vi "Main.vi"(11 "Module Admin":refnum<class "Delacor_lib_QMH_Module Admin.lvclass">) -> ()   [LabVIEW 2019, in "MAIN.lvlib"]
doc: "This template is based off of the Queued Message Handler design pattern and the Queued Message Handler project template that ships with LabVIEW.\n\nThe main difference is that the queue is private to this module and communication between modules is performed via Broadcast and Request events.\n\nRequest events are wrapped in public API methods and are handled in the Event Handling Loop (EHL) of this VI. Any module can register for Broadcast events sent by this module. The EHL generates messages based on user interface actions.\n\nThe Message Handling Loop (MHL) processes messages generated by the EHL, or by other messages. The messages are string values, so new messages can be added easily to the Message Cases case structure in the MHL. Each message cluster can also provide an optional value for Message Data, which is a variant that can be converted to whatever message-specific data is required.\n_____\nBased on Delacor QMH Project Template 5.0.0.82."
uses:
  MAIN.lvlib
  <vilib>/Delacor/Delacor QMH/Libraries/Module Admin_class/Delacor_lib_QMH_Module Admin.lvclass
  Module Data--cluster.ctl
  <vilib>/Delacor/Delacor QMH/Libraries/Message Queue_class/Delacor_lib_QMH_Message Queue.lvclass/Delacor_lib_QMH_Message Queue.ctl
  Stop Argument--cluster.ctl
  <vilib>/Delacor/Delacor QMH/Libraries/Module Admin_class/Delacor_lib_QMH_Module Admin.lvclass/Delacor_lib_QMH_Module Admin.ctl
  START HELPER LOOP Argument--cluster.ctl
  STOP HELPER LOOP Argument--cluster.ctl
  SOLICITAR DATOS DE CONEXION Argument--cluster.ctl
  <vilib>/Utility/miscctls.llb/LVPointTypeDef.ctl
  <vilib>/Delacor/Delacor QMH/Libraries/Message Queue_class/Delacor_lib_QMH_Enqueue Message (Single).vi
  <vilib>/Delacor/Delacor QMH/Libraries/Module Admin_class/Delacor_lib_QMH_Get External Launch.vi
  <vilib>/Utility/error.llb/Error Cluster From Error Code.vi
  <vilib>/ErrorRing/Error Ring.xnode
  <vilib>/Delacor/Delacor QMH/Libraries/Message Queue_class/Delacor_lib_QMH_Message Queue.lvclass
panel:
  out "Microcontrolador":string
  out "SE CONECTÓ?":bool
  in  "CONECTAR AL MICRO":bool
  in  "PUERTO DE CONEXIÓN":refnum<visa-resource-name>
  in  "Simulate MHL Error":bool
  in  "Simulate EHL Error":bool
  out "error out":errorcluster
  out "Status":string
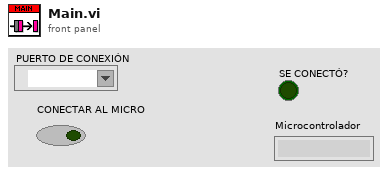
[diagram p1: front panel]
types:
  T1 = typedef "MAIN.lvlib/Request Events--cluster.ctl" = cluster{"Stop Module":refnum<user-event>, "Show Panel":refnum<user-event>, "Hide Panel":refnum<user-event>, "Get Module Execution Status":refnum<user-event>, "Show Diagram":refnum<user-event>, "START HELPER LOOP":refnum<user-event>, "STOP HELPER LOOP":refnum<user-event>, "SOLICITAR DATOS DE CONEXION":refnum<user-event>}
  T2 = typedef "CONEXIÓN CON EL MICRO.lvlib/Broadcast Events--cluster.ctl" = cluster{"Module Did Init":refnum<user-event>, "Status Updated":refnum<user-event>, "Error Reported":refnum<user-event>, "Module Did Stop":refnum<user-event>, "Update Module Execution Status":refnum<user-event>}
  T3 = typedef "MAIN.lvlib/Module Data--cluster.ctl" = cluster{"Status":string}
  T4 = enum32{"invalid lock state", "Not Locked", "Locked (No Password)", "Password-protected"}
  T5 = typedef "MAIN.lvlib/Stop Argument--cluster.ctl" = cluster{"Origin":string, "Exit via Stop Module Req?":bool, "Wait for Module to stop?":bool}
  T6 = typedef "MAIN.lvlib/START HELPER LOOP Argument--cluster.ctl" = cluster{"DELAY TIMEOUT":i32}
  T7 = typedef "MAIN.lvlib/STOP HELPER LOOP Argument--cluster.ctl" = cluster{"Boolean":bool}
  T8 = typedef "MAIN.lvlib/SOLICITAR DATOS DE CONEXION Argument--cluster.ctl" = cluster{"VISA resource name":refnum<visa-resource-name>, "ESTADO ERROR":string, "SE CONECTÓ?":bool, "MICRO":string}
  T9 = typedef "LVPointTypeDef.ctl" = cluster{"Horizontal":i16, "Vertical":i16}
  T10 = enum32{"Invalid", "Standard", "Closed", "Hidden", "Minimized", "Maximized"}
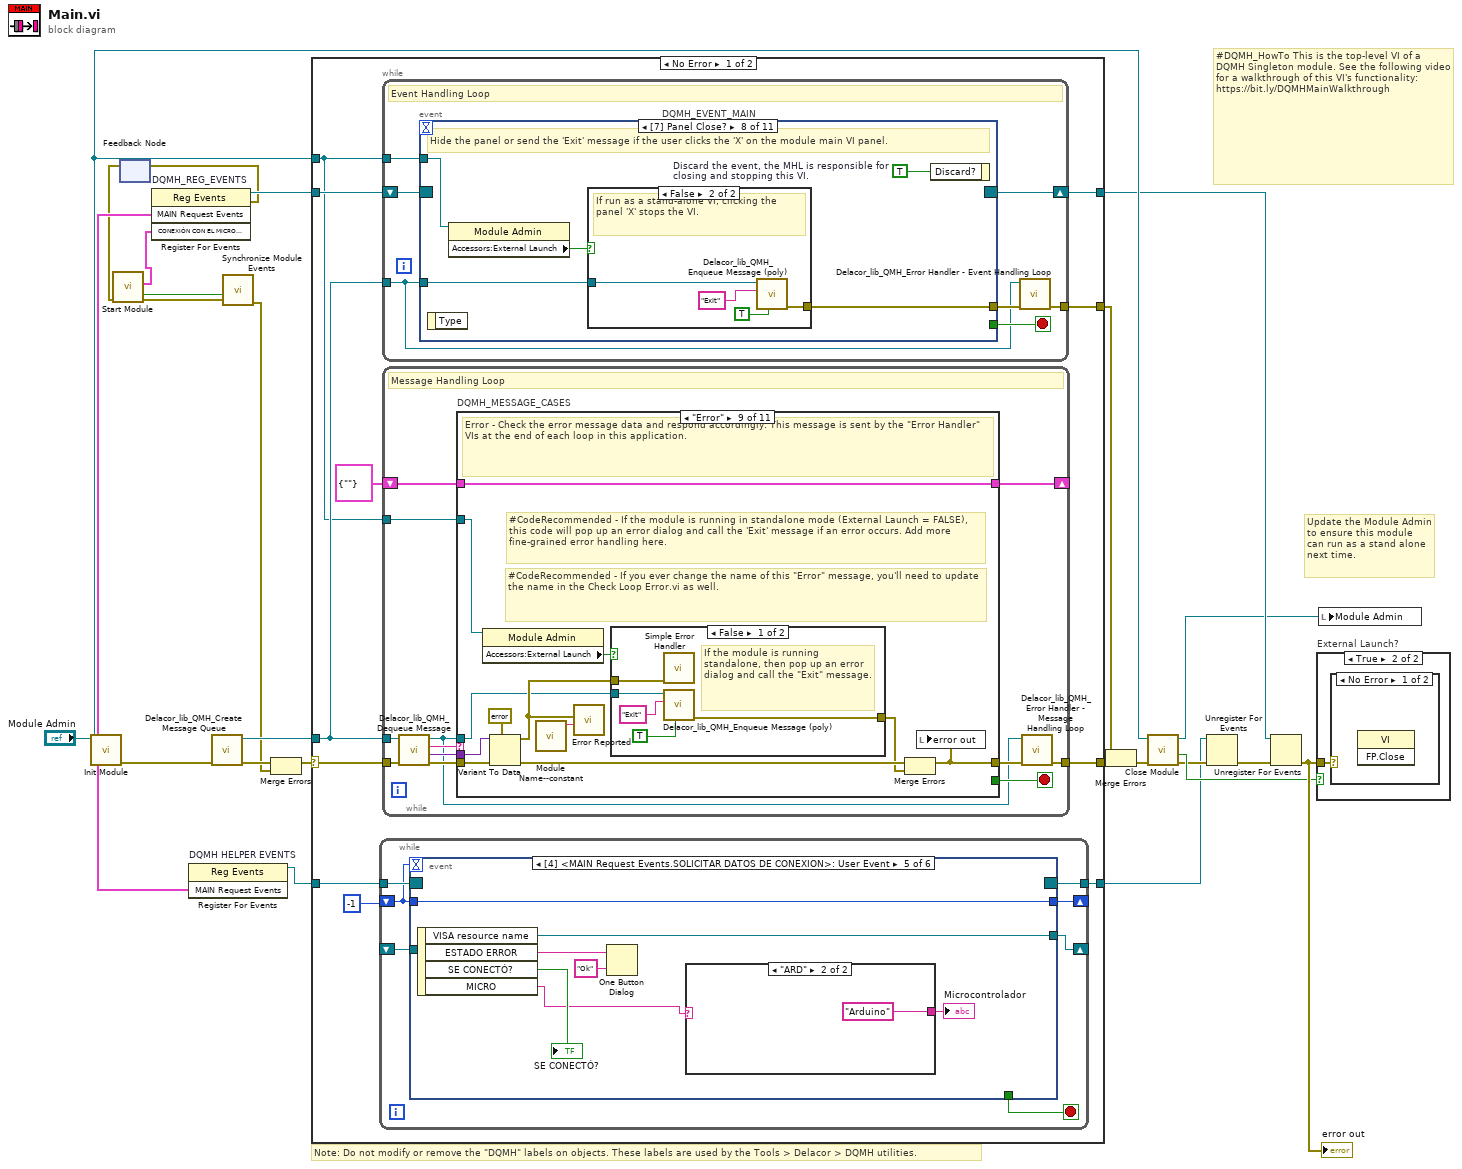
[diagram p0: block diagram]
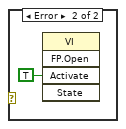
[diagram p3: hidden frame]
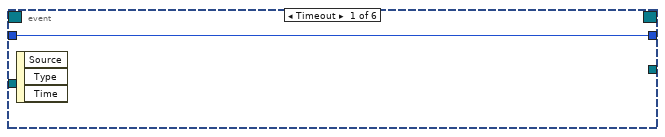
[diagram p4: hidden frame]
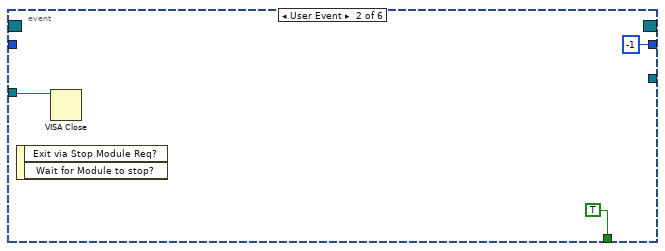
[diagram p5: hidden frame]
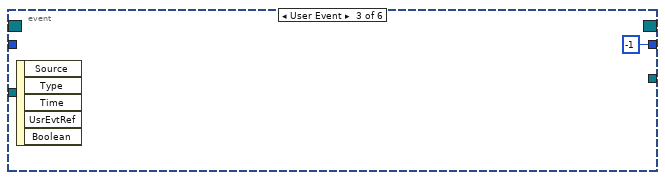
[diagram p6: hidden frame]
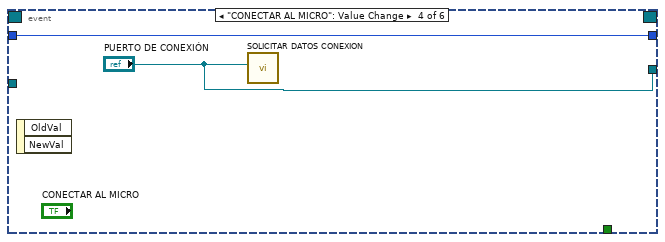
[diagram p7: hidden frame]
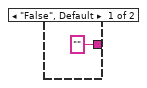
[diagram p8: hidden frame]
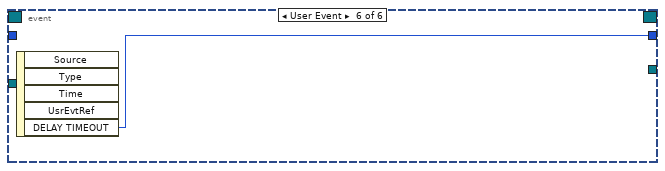
[diagram p9: hidden frame]
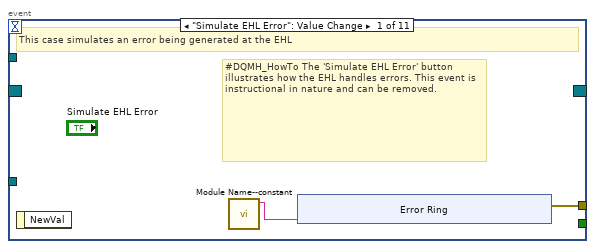
[diagram p10: hidden frame]
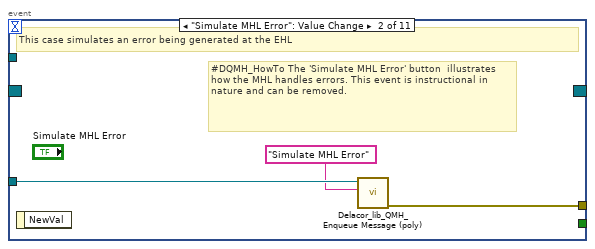
[diagram p11: hidden frame]
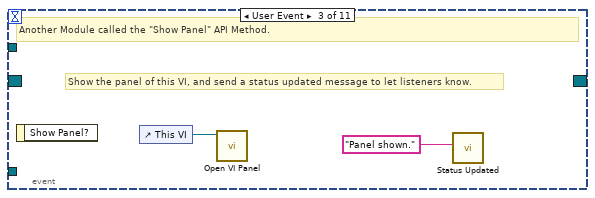
[diagram p12: hidden frame]
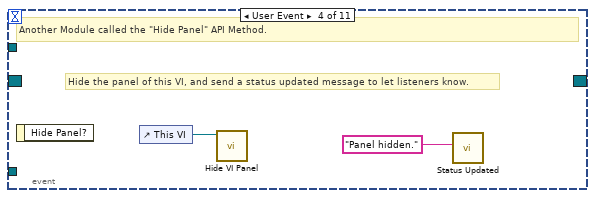
[diagram p13: hidden frame]
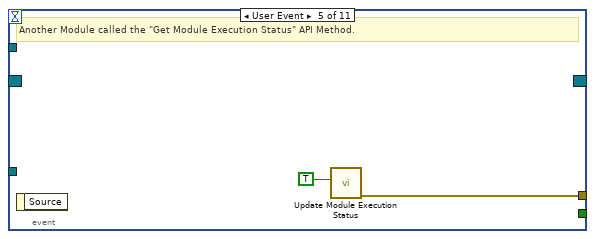
[diagram p14: hidden frame]
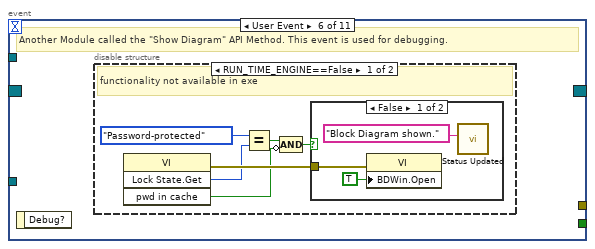
[diagram p15: hidden frame]
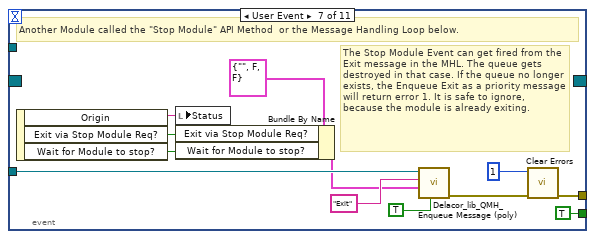
[diagram p18: hidden frame]
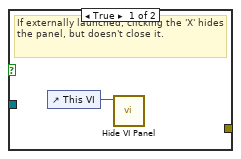
[diagram p19: hidden frame]
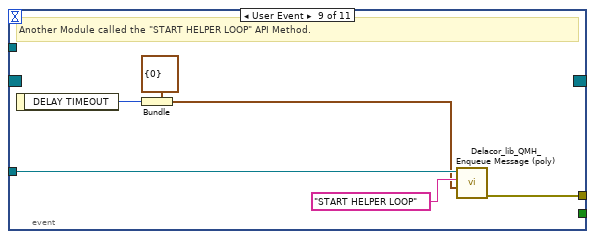
[diagram p20: hidden frame]
diagram:
  # "#DQMH_HowTo This is the top-level VI of a DQMH Singleton module. See the following video for a walkthrough of this VI's functionality: https://bit.ly/DQMHMainWalkthrough"
  # "Note: Do not modify or remove the \"DQMH\" labels on objects. These labels are used by the Tools > Delacor > DQMH utilities."
  # "Update the Module Admin to ensure this module can run as a stand alone next time."
  n1 = call "Init Module.vi"("Singleton Module Admin in"="Module Admin") -> ("error out"=w24:errorcluster, "MAIN Request Events"=w8:T1, "Singleton Module Admin out"=w18:refnum<class "Delacor_lib_QMH_Module Admin.lvclass">)  [unwired: 8 in]
  n2 = feedback #1() -> (w1:errorcluster)  [unwired: 1 in]
  n3 = call "Start Module.vi"("error in (no error)"=w1) -> ("error out"=w4:errorcluster, "Wait for Event Sync?"=w5:bool, "CONEXIÓN CON EL MICRO Broadcast Events"=w6:T2)  [unwired: 7 in, 1 out]
  n4 = register-events "DQMH_REG_EVENTS"(w8, w6) -> (reference out=w16:refnum<event-registration>, error out=w2:errorcluster)  [unwired: 2 in]
  n5 = feedback-in #1(w2) -> ()
  n6 = register-events "DQMH HELPER EVENTS"(w8) -> (reference out=w7:refnum<event-registration>)  [unwired: 2 in, 1 out]
  n7 = call <vilib>:"Delacor_lib_QMH_Create Message Queue.vi"("error in (no error)"=w24) -> ("error out"=w20:errorcluster, "Message Queue"=w15:refnum<class "Delacor_lib_QMH_Message Queue.lvclass">)  [unwired: 9 in]
  n8 = call "Synchronize Module Events.vi"("error in (no error)"=w4, "Wait for Event Sync?"=w5) -> ("error out"=w3:errorcluster)  [unwired: 9 in]
  n9 = Merge Errors(w20, w3) -> (w19:errorcluster)
  n10 = case shown="No Error" w19 {
    selector: w19 -> [w34 w256]
    tunnel: [w36 w255] -> w25
    tunnel: [w33 w261] -> w17
    tunnel: w16 -> [w31 w261]
    tunnel: w15 -> [w30 w254]
    tunnel: [w35 _] -> w23
    tunnel: w18 -> [w29 w257]
    tunnel: [w28 w253] -> w9
    tunnel: w7 -> [w27 w253]
    frame No Error {
      n11 = while {
        tunnel: [w43] -> w28
        tunnel: w27 -> [w42]
        shift-right: [w41] -> _
        shift-left: -1 -> [w40]
        shift-right: [w38] -> _
        shift-left: _ -> [w37]
        stop <- w39 stop-if-true
        n12 = event shown="[4] <MAIN Request Events.SOLICITAR DATOS DE CONEXION>: User Event" {
          selector: w42 -> [_ _ _ _ _ _]
          dyn-events: [_ _ _ _ _ _] -> w43
          timeout: w40 -> [_ _ _ _ _ _]
          tunnel: [w44 -1 ("DELAY TIMEOUT") -1 ("DELAY TIMEOUT") w50 w57 w60] -> w41
          tunnel: w40 -> [w44 _ _ w50 w57 _]
          tunnel: [_ TRUE _ _ _ _] -> w39
          tunnel: [_ _ _ "PUERTO DE CONEXIÓN" w56 _] -> w38
          tunnel: w37 -> [_ w45 _ _ _ _]
          event Timeout {
            n13 = event-data() -> ()  [unwired: 1 in, 3 out]
          }
          event User Event {
            n14 = event-data() -> ()  [unwired: 1 in, 2 out]
            n15 = VISA Close(VISA resource name=w45) -> ()  [unwired: 1 in, 1 out]
          }
          event User Event {
            n16 = event-data() -> ()  [unwired: 1 in, 5 out]
          }
          event "CONECTAR AL MICRO": Value Change {
            n17 = event-data() -> ()  [unwired: 1 in, 2 out]
            n18 = call "SOLICITAR DATOS CONEXION.vi"("VISA resource name"="PUERTO DE CONEXIÓN") -> ()  [unwired: 10 in, 1 out]
          }
          event User Event {
            n19 = event-data() -> ("VISA resource name"=w56:refnum<visa-resource-name>, "ESTADO ERROR"=w55:string, "SE CONECTÓ?"=→"SE CONECTÓ?":bool, "MICRO"=w52:string)  [unwired: 1 in]
            n20 = One Button Dialog(message=w55, button name ("OK")="Ok") -> ()  [unwired: 1 out]
            n21 = case shown="\"ARD\"" w52 {
              tunnel: ["" "Arduino"] -> w51
              frame "False", Default {
              }
              frame "ARD" {
              }
            }
            "Microcontrolador" <- w51
          }
          event User Event {
            n22 = event-data() -> ("DELAY TIMEOUT"=w60:i32)  [unwired: 1 in, 4 out]
          }
        }
      }
      n23 = while {
        tunnel: w30 -> [w61]
        shift-right: [w64] -> w33
        shift-left: w31 -> [w65]
        tunnel: [w66] -> w35
        tunnel: w29 -> [w62]
        stop <- w63 stop-if-true
        # "Event Handling Loop"
        n24 = event "DQMH_EVENT_MAIN" shown="[7] Panel Close?" {
          selector: w65 -> [_ _ _ _ _ _ _ _ _ _ _]
          dyn-events: [_ _ _ _ _ _ _ _ _ _ _] -> w64
          timeout: _ -> [_ _ _ _ _ _ _ _ _ _ _]
          tunnel: [_ _ _ _ _ _ TRUE ("Discard?") _ _ _ _] -> w63
          tunnel: w61 -> [_ w78 _ _ _ _ w102 w109 w122 w128 w137]
          tunnel: [w69 w79 _ _ w85 _ w105 w111 w117 w123 w129] -> w67
          tunnel: w62 -> [_ _ _ _ _ _ _ w108 _ _ _]
          event "Simulate EHL Error": Value Change {
            # "#DQMH_HowTo The 'Simulate EHL Error' button  illustrates how the EHL handles errors. This event is instructional in nature and can be removed."
            # "This case simulates an error being generated at the EHL"
            n25 = event-data() -> ()  [unwired: 1 in, 1 out]
            n26 = call "Module Name--constant.vi"() -> ("Module Name"=w68:string)  [unwired: 11 in]
            n27 = xnode "Error Ring"("parameter 0"=w68) -> ("error out"=w69:errorcluster)
          }
          event "Simulate MHL Error": Value Change {
            # "#DQMH_HowTo The 'Simulate MHL Error' button  illustrates how the MHL handles errors. This event is instructional in nature and can be removed."
            # "This case simulates an error being generated at the EHL"
            n28 = event-data() -> ()  [unwired: 1 in, 1 out]
            n29 = call-poly <vilib>:"Delacor_lib_QMH_Enqueue Message (poly).vi"("Message"="Simulate MHL Error", "Message Queue in"=w78) -> ("error out"=w79:errorcluster)  [unwired: 8 in, 1 out]
          }
          event User Event {
            # "Show the panel of this VI, and send a status updated message to let listeners know."
            # "Another Module called the \"Show Panel\" API Method."
            n30 = event-data() -> ()  [unwired: 1 in, 1 out]
            n31 = control-ref of="This VI"() -> (w81:refnum<vi>)
            n32 = call "Open VI Panel.vi"("VI"=w81) -> ()  [unwired: 10 in, 1 out]
            n33 = call "Status Updated.vi"("Status"="Panel shown." ("format string")) -> ()  [unwired: 10 in, 1 out]
          }
          event User Event {
            # "Hide the panel of this VI, and send a status updated message to let listeners know."
            # "Another Module called the \"Hide Panel\" API Method."
            n34 = event-data() -> ()  [unwired: 1 in, 1 out]
            n35 = control-ref of="This VI"() -> (w83:refnum<vi>)
            n36 = call "Hide VI Panel.vi"("VI"=w83) -> ()  [unwired: 10 in, 1 out]
            n37 = call "Status Updated.vi"("Status"="Panel hidden." ("format string")) -> ()  [unwired: 10 in, 1 out]
          }
          event User Event {
            # "Another Module called the \"Get Module Execution Status\" API Method."
            n38 = event-data() -> ()  [unwired: 1 in, 1 out]
            n39 = call "Update Module Execution Status.vi"("Running?"=TRUE) -> ("error out"=w85:errorcluster)  [unwired: 10 in]
          }
          event User Event {
            # "Another Module called the \"Show Diagram\" API Method. This event is used for debugging."
            n40 = event-data() -> ()  [unwired: 1 in, 1 out]
            n41 = disable-structure shown="RUN_TIME_ENGINE==False" {
              frame condition #0 (active) {
                # "functionality not available in exe"
                n42 = invoke class="VI" method="Lock State.Get"() -> (error out=w91:errorcluster, "Get Lock State"=w90:T4, "pwd in cache"=w87:bool)  [unwired: 4 in, 1 out]
                n43 = Equal?(x=T4."Password-protected", y=w90) -> (x = y?=w88:bool)
                n44 = Compound Arithmetic op=AND(w88, invert w87) -> (w86:bool)
                n45 = case shown="False" w86 {
                  tunnel: w91 -> [w94 _]
                  frame False {
                    n46 = property class="VI"(error in=w94, "BDWin.Open"=TRUE ("Block Diagram Window:Open")) -> ()  [unwired: 1 in, 2 out]
                    n47 = call "Status Updated.vi"("Status"="Block Diagram shown." ("format string")) -> ()  [unwired: 10 in, 1 out]
                  }
                  frame True {
                    # "Password-protected VI, and the password is not in the cache. Do not show the diagram."
                  }
                }
              }
              frame condition #1 {
              }
            }
          }
          event User Event {
            # "The Stop Module Event can get fired from the Exit message in the MHL. The queue gets destroyed in that case. If the queue no longer exists, the Enqueue Exit as a priority message will return error 1. It is safe to ignore, because the module is already exiting."
            # "Another Module called the \"Stop Module\" API Method  or the Message Handling Loop below."
            n48 = event-data() -> ("Origin"=w101:string, "Exit via Stop Module Req?"=w97:bool, "Wait for Module to stop?"=w96:bool)  [unwired: 1 in]
            n49 = local write "Status"(w101) -> ()
            n50 = Bundle By Name(cluster=T5 {"Origin"="", "Exit via Stop Module Req?"=FALSE, "Wait for Module to stop?"=FALSE} ("Stop Argument"), "Exit via Stop Module Req?"=w97, "Wait for Module to stop?"=w96) -> (w95:T5)
            n51 = call-poly <vilib>:"Delacor_lib_QMH_Enqueue Message (poly).vi"("Priority Message? (F)"=TRUE, "Message Data"=w95, "Message"="Exit", "Message Queue in"=w102) -> ("error out"=w106:errorcluster)  [unwired: 6 in, 1 out]
            n52 = call <vilib>:"Clear Errors.vi"("error in (no error)"=w106, "specific error code to clear (0: all)"=1) -> ("error out"=w105:errorcluster)  [unwired: 4 in, 1 out]
          }
          event Panel Close? {
            w110 = TRUE  # Discard the event, the MHL is responsible for closing and stopping this VI.
            # "Hide the panel or send the 'Exit' message if the user clicks the 'X' on the module main VI panel."
            n53 = event-data() -> ()  [unwired: 1 in, 1 out]
            n54 = property class="Module Admin"(reference=w108) -> ("Accessors:External Launch"=w107:bool)  [unwired: 1 in, 2 out]
            n55 = case shown="False" w107 {
              tunnel: w109 -> [_ w115]
              tunnel: [_ w116] -> w111
              frame True {
                # "If externally launched, clicking the 'X' hides the panel, but doesn't close it."
                n56 = control-ref of="This VI"() -> (w112:refnum<vi>)
                n57 = call "Hide VI Panel.vi"("VI"=w112) -> ()  [unwired: 10 in, 1 out]
              }
              frame False {
                # "If run as a stand-alone VI, clicking the panel 'X' stops the VI."
                n58 = call-poly <vilib>:"Delacor_lib_QMH_Enqueue Message (poly).vi"("Priority Message? (F)"=TRUE, "Message"="Exit", "Message Queue in"=w115) -> ("error out"=w116:errorcluster)  [unwired: 7 in, 1 out]
              }
            }
            n59 = event-data("Discard?"=w110) -> ()  [unwired: 1 in, 1 out]
          }
          event User Event {
            # "Another Module called the \"START HELPER LOOP\" API Method."
            n60 = event-data() -> ("DELAY TIMEOUT"=w118:i32)  [unwired: 1 in]
            n61 = Bundle(cluster=T6 {"DELAY TIMEOUT"=0} ("START HELPER LOOP Argument"), "DELAY TIMEOUT"=w118) -> (w119:T6)
            n62 = call-poly <vilib>:"Delacor_lib_QMH_Enqueue Message (poly).vi"("Message Data"=w119, "Message"="START HELPER LOOP", "Message Queue in"=w122) -> ("error out"=w117:errorcluster)  [unwired: 7 in, 1 out]
          }
          event User Event {
            # "Another Module called the \"STOP HELPER LOOP\" API Method."
            n63 = event-data() -> ("Boolean"=w124:bool)  [unwired: 1 in]
            n64 = Bundle(cluster=T7 {"Boolean"=FALSE} ("STOP HELPER LOOP Argument"), "Boolean"=w124) -> (w125:T7)
            n65 = call-poly <vilib>:"Delacor_lib_QMH_Enqueue Message (poly).vi"("Message Data"=w125, "Message"="STOP HELPER LOOP", "Message Queue in"=w128) -> ("error out"=w123:errorcluster)  [unwired: 7 in, 1 out]
          }
          event User Event {
            # "Another Module called the \"SOLICITAR DATOS DE CONEXION\" API Method."
            n66 = event-data() -> ("VISA resource name"=w133:refnum<visa-resource-name>, "ESTADO ERROR"=w132:string, "SE CONECTÓ?"=w131:bool, "MICRO"=w130:string)  [unwired: 1 in]
            n67 = Bundle(cluster=T8 {"VISA resource name"="", "ESTADO ERROR"="", "SE CONECTÓ?"=FALSE, "MICRO"=""} ("SOLICITAR DATOS DE CONEXION Argument"), "VISA resource name"=w133, "ESTADO ERROR"=w132, "SE CONECTÓ?"=w131, "MICRO"=w130) -> (w134:T8)
            n68 = call-poly <vilib>:"Delacor_lib_QMH_Enqueue Message (poly).vi"("Message Data"=w134, "Message"="SOLICITAR DATOS DE CONEXION", "Message Queue in"=w137) -> ("error out"=w129:errorcluster)  [unwired: 7 in, 1 out]
          }
        }
        n69 = call-dynamic "Delacor_lib_QMH_Error Handler - Event Handling Loop.vi"("error in (no error)"=w67, "Message Queue in"=w61) -> ("dup error in"=w66:errorcluster)  [unwired: 8 in, 1 out]
      }
      n70 = while {
        tunnel: w30 -> [w140]
        shift-right: [w144] -> _
        shift-left: T3 {"Status"=""} ("Data Cluster") -> [w145]
        tunnel: w34 -> [w148]
        tunnel: [w146] -> w36
        tunnel: w29 -> [w138]
        stop <- w143 stop-if-true
        # "Message Handling Loop"
        n71 = call-dynamic "Delacor_lib_QMH_Dequeue Message.vi"("error in (no error)"=w148, "Message Queue in"=w140) -> ("error out"=w147:errorcluster, "Message Data"=w141:variant, "Message"=w142:string, "Message Queue out"=w139:refnum<class "Delacor_lib_QMH_Message Queue.lvclass">)  [unwired: 6 in]
        n72 = case "DQMH_MESSAGE_CASES" shown="\"Error\"" w142 {
          selector: w142 -> [_ _ _ _ _ _ _ _ _ _ w240]
          tunnel: w139 -> [_ _ _ _ _ _ _ _ w210 w232 _]
          tunnel: w147 -> [w167 w171 w177 w183 w189 w192 w194 w199 w217 w238 w242]
          tunnel: [w165 w171 w175 w181 w187 w191 w194 w198 w213 w235 w243] -> w149
          tunnel: w145 -> [w156 w170 w176 w182 w188 w190 w193 w196 w212 w231 w241]
          tunnel: [w155 w170 w176 w182 w188 w190 w193 w196 w212 w231 w241] -> w144
          tunnel: [_ _ _ _ _ _ _ _ _ w230 _] -> w143
          tunnel: w141 -> [_ _ w174 w180 w186 _ _ _ w211 w229 _]
          tunnel: w138 -> [w157 _ _ _ _ _ _ _ w209 w224 _]
          frame "Initialize" {
            w150 = "Initial Message" ("Initial Message")
            # "#CodeNeeded - Initialize the appearance of the front panel."
            # "#CodeNeeded - Initialize your state data here."
            # "Initialize - Any operation that needs to be done before the module can receive messages. Synchronize Caller Events.vi will inform Start Module.vi that the module has launched and is ready to receive messages. Module Did Init.vi will broadcast that the module initialized."
            n73 = call "Synchronize Caller Events.vi"("error in (no error)"=w167, "Singleton Module Admin in"=w157) -> ("error out"=w166:errorcluster, "Singleton Module Admin out"=w152:refnum<class "Delacor_lib_QMH_Module Admin.lvclass">)  [unwired: 8 in]
            n74 = property class="Module Admin"(reference=w152) -> ("Accessors:External Launch"=w161:bool)  [unwired: 1 in, 2 out]
            n75 = Select(t=T10."Hidden" ("State"), s=w161, f=T10."Standard" ("State")) -> (s? t:f=w158:T10)
            n76 = call "Module Name--constant.vi"() -> ("Module Name"=w164:string)  [unwired: 11 in]
            n77 = property class="VI"("Front Panel.Title"=w164) -> (reference out=w163:refnum<vi>, error out=w169:errorcluster)  [unwired: 2 in]
            n78 = call "Module Name--constant.vi"() -> ("Module Name"=w153:string)  [unwired: 11 in]
            n79 = invoke class="VI" method="FP.Open"(reference=w163, error in=w169, "State"=w158) -> (reference out=w162:refnum<vi>, error out=w168:errorcluster)  [unwired: 2 in, 3 out]
            n80 = Bundle By Name(cluster=w156, "Status"=w150) -> (w155:T3)
            n81 = call "Module Did Init.vi"("error in (no error)"=w166, "Initialized?"=TRUE, "Origin"=w153) -> ("error out"=w165:errorcluster)  [unwired: 8 in]
            n82 = invoke class="VI" method="FP.Center"(reference=w162, error in=w168) -> ()  [unwired: 1 in, 3 out]
            n83 = property on="Pane" class="Pane"("Origin"=T9 {"Horizontal"=0, "Vertical"=0}) -> ()  [unwired: 2 in, 2 out]
            "Status" <- w150
          }
          frame "--- Module Specific ---" {
            # "Separator -- The following cases handle messages specific to this Module."
          }
          frame "START HELPER LOOP" {
            # "#CodeNeeded\n1. Configure this Message Case for handling the \"START HELPER LOOP\" message.\n2. Delete or edit this label when done."
            # "INICIALIZAR HELPER LOOP"
            n84 = Variant To Data(error in=w177, type=T6 {"DELAY TIMEOUT"=0} ("START HELPER LOOP Argument"), Variant=w174) -> (data=w172:T6, error out=w175:errorcluster)
            n85 = Unbundle By Name(w172) -> ()  [unwired: 1 out]
          }
          frame "STOP HELPER LOOP" {
            # "#CodeNeeded\n1. Configure this Message Case for handling the \"STOP HELPER LOOP\" message.\n2. Delete or edit this label when done."
            # "STOP HELPER LOOP"
            n86 = Variant To Data(error in=w183, type=T7 {"Boolean"=FALSE} ("STOP HELPER LOOP Argument"), Variant=w180) -> (data=w178:T7, error out=w181:errorcluster)
            n87 = Unbundle By Name(w178) -> ()  [unwired: 1 out]
          }
          frame "SOLICITAR DATOS DE CONEXION" {
            # "#CodeNeeded\n1. Configure this Message Case for handling the \"SOLICITAR DATOS DE CONEXION\" message.\n2. Delete or edit this label when done."
            # "EL MAIN SOLICITA AL MODULO DE CONEXIÓN QUE LE MANDE LAS SIGUIENTES COSAS:\nSESIÓN DE LA CONEXIÓN\nESTADO CONEXIÓN \nESTADO DE ERRORES\nA QUE MICROCONTROLADOR SE CONECTÓ"
            n88 = Variant To Data(error in=w189, type=T8 {"VISA resource name"="", "ESTADO ERROR"="", "SE CONECTÓ?"=FALSE, "MICRO"=""} ("SOLICITAR DATOS DE CONEXION Argument"), Variant=w186) -> (data=w184:T8, error out=w187:errorcluster)
            n89 = Unbundle By Name(w184) -> ()  [unwired: 4 out]
          }
          frame "---Copy This Frame---" {
            # "Duplicate this frame when creating new messages.  Change this comment in the duplicated frame to describe this message."
            n90 = Merge Errors(w192) -> (w191:errorcluster)
          }
          frame "--- Exit and Error Handling---" {
            # "Separator - The following cases handle errors and exit messages."
          }
          frame "Simulate MHL Error" {
            # "#DQMH_HowTo The 'Simulate MHL Error' button  illustrates how the MHL handles errors. This event is instructional in nature and can be removed."
            # "Simulate an error occurring at the MHL"
            n91 = call "Module Name--constant.vi"() -> ("Module Name"=w195:string)  [unwired: 11 in]
            n92 = xnode "Error Ring"("parameter 0"=w195) -> ("error out"=w197:errorcluster)
            n93 = Merge Errors(w199, w197) -> (w198:errorcluster)
          }
          frame "Error" {
            # "#CodeRecommended - If you ever change the name of this \"Error\" message, you'll need to update the name in the Check Loop Error.vi as well."
            # "#CodeRecommended - If the module is running in standalone mode (External Launch = FALSE), this code will pop up an error dialog and call the 'Exit' message if an error occurs. Add more fine-grained error handling here."
            # "Error - Check the error message data and respond accordingly. This message is sent by the \"Error Handler\" VIs at the end of each loop in this application."
            n94 = property class="Module Admin"(reference=w209) -> ("Accessors:External Launch"=w208:bool)  [unwired: 1 in, 2 out]
            n95 = Variant To Data(error in=w217, type=errorcluster {"status"=FALSE, "code"=0, "source"=""} ("error constant"), Variant=w211) -> (data=w218:errorcluster, error out=w215:errorcluster)
            n96 = call "Module Name--constant.vi"() -> ("Module Name"=w207:string)  [unwired: 11 in]
            n97 = call "Error Reported.vi"("Additional Information"=w207, "Error"=w218) -> ()  [unwired: 9 in, 1 out]
            n98 = case shown="False" w208 {
              tunnel: [w223 _] -> w214
              tunnel: w210 -> [w221 _]
              tunnel: w218 -> [w222 _]
              frame False {
                # "If the module is running standalone, then pop up an error dialog and call the \"Exit\" message."
                n99 = call <vilib>:"Simple Error Handler.vi"("error in (no error)"=w222) -> ()  [unwired: 4 in, 5 out]
                n100 = call-poly <vilib>:"Delacor_lib_QMH_Enqueue Message (poly).vi"("Priority Message? (F)"=TRUE, "Message"="Exit", "Message Queue in"=w221) -> ("error out"=w223:errorcluster)  [unwired: 7 in, 1 out]
              }
              frame True {
                # "If the module was launched externally, calling the Error Reported broadcast VI is the only action performed by the \"Error\" message. The module's caller can then process the error appropriately."
              }
            }
            n101 = Merge Errors(w215, w214) -> (w213:errorcluster)
            n102 = local write "error out"(w213) -> ()
          }
          frame "Exit" {
            w228 = 91  # 91: not all Exit messages will have an argument
            w230 = TRUE  # Stop the VI
            # "Release the message queue reference"
            # "#CodeNeeded - Add any required cleanup code here"
            # "Exit - Exit the application."
            n103 = Variant To Data(error in=w238, type=T5 {"Origin"="", "Exit via Stop Module Req?"=FALSE, "Wait for Module to stop?"=FALSE} ("Stop Argument"), Variant=w229) -> (data=w226:T5, error out=w234:errorcluster)
            n104 = call <vilib>:"Clear Errors.vi"("error in (no error)"=w234, "specific error code to clear (0: all)"=w228) -> ("error out"=w237:errorcluster)  [unwired: 4 in, 1 out]
            n105 = control-ref of="This VI"() -> (w225:refnum<vi>)
            n106 = call-dynamic "Delacor_lib_QMH_Release Message Queue.vi"("error in (no error)"=w237, "Message Queue"=w232) -> ("error out"=w236:errorcluster)  [unwired: 9 in]
            n107 = call "Handle Exit.vi"("Stop Argument"=w226, "Admin in"=w224, "VI reference"=w225) -> ("error out"=w233:errorcluster)  [unwired: 7 in, 1 out]
            n108 = Merge Errors(w236, w233) -> (w235:errorcluster)
          }
          frame Default {
            # "'Default' case only runs if there is a message that isn't defined in any of the other cases.  Output a programming error."
            n109 = call "Module Name--constant.vi"() -> ("Module Name"=w239:string)  [unwired: 11 in]
            n110 = xnode "Error Ring"("parameter 0"=w240, "parameter 1"=w239) -> ("error out"=w244:errorcluster)
            n111 = Merge Errors(w242, w244) -> (w243:errorcluster)
          }
        }
        n112 = call-dynamic "Delacor_lib_QMH_Error Handler - Message Handling Loop.vi"("error in (no error)"=w149, "Message Queue in"=w139) -> ("dup error in"=w146:errorcluster)  [unwired: 8 in, 1 out]
      }
    }
    frame Error {
      # "Synchronize Caller Events.vi will inform Start Module.vi that the module has launched and will let the code calling Start Module.vi register for broadcasts and would permit the caller receive the broadcast that an error occurred at launch time."
      n113 = call-dynamic "Delacor_lib_QMH_Release Message Queue.vi"("error in (no error)"=w256, "Message Queue"=w254) -> ("error out"=w255:errorcluster)  [unwired: 9 in]
      n114 = call "Synchronize Caller Events.vi"("Singleton Module Admin in"=w257) -> ("error out"=w262:errorcluster)  [unwired: 9 in, 1 out]
      n115 = call "Module Name--constant.vi"() -> ("Module Name"=w260:string)  [unwired: 11 in]
      n116 = Format Into String(format string="An error occurred during initialization. %s is no longer running.", w260) -> (resulting string=w258:string)  [unwired: 2 in, 1 out]
      n117 = Merge Errors(w255, w262) -> (w263:errorcluster)
      n118 = call "Error Reported.vi"("Additional Information"=w258, "Error"=w263) -> ()  [unwired: 9 in, 1 out]
    }
  }
  n119 = Merge Errors(w23, w25) -> (w22:errorcluster)
  n120 = call "Close Module.vi"("error in (no error)"=w22, "Module Admin in"=w18) -> ("error out"=w10:errorcluster, "External Launch"=w12:bool, "Module Admin out"=w13:refnum<class "Delacor_lib_QMH_Module Admin.lvclass">)  [unwired: 7 in]
  n121 = Unregister For Events(event registration refnum=w9, error in=w10) -> (error out=w11:errorcluster)
  n122 = Unregister For Events(event registration refnum=w17, error in=w11) -> (error out=w21:errorcluster)
  "error out" <- w21
  n123 = case "External Launch?" shown="True" w12 {
    tunnel: w21 -> [_ w264]
    frame False {
    }
    frame True {
      n124 = case shown="No Error" w264 {
        frame No Error {
          n125 = invoke class="VI" method="FP.Close"() -> ()  [unwired: 3 in, 3 out]
        }
        frame Error {
          n126 = invoke class="VI" method="FP.Open"("Activate"=TRUE ("Activate?")) -> ()  [unwired: 4 in, 5 out]
        }
      }
    }
  }
  n127 = local write "Module Admin"(w13) -> ()
